vi "24_1.vi"() -> ()   [LabVIEW 2020]
panel:
  out "sum":i16=10
  in  "Switch":bool=TRUE
  in  "Input":string="nwneswnwnwsenwnwnwnwnwnwnwnwnwnenwnwnwnw\nseseswswseseswsesenwnwseseswsese\nswneeweneeneneeneeeeeneeeene\neswswnwswswwnwswswswswewswswswswswsw\nwwseneseeneseswwwseneseseneswseswese\nseseseswseseseseswnwswswneseseswsesesese\nnwnewwwwwswnwnwww\nneesenwwswseswswswnwsenwsesewseeeswse\nsweeneesweeswnweewseeneeneneswnw\nswseswseswswseseswseneswseswswsesesesese\nswneneneenenenenenenenenenenenwne\nswswswswswswswswswswswesenwseswswswse\nneeeenweneeneswene\nswwnenwsewwwswswwswwswweewwswwnw\nenewwnenwnenenenwnewnenenwnenenenwee\nnwwnwnwnwnwnwnwenewnwsenwwwwwnwswnw\neeenweeeesweeeneeseeeeswee\nwswwswseswwswswwwnww\nswenwwn..."
  in  "Input Test":string="sesenwnenenewseeswwswswwnenewsewsw\nneeenesenwnwwswnenewnwwsewnenwseswesw\nseswneswswsenwwnwse\nnwnwneseeswswnenewneswwnewseswneseene\nswweswneswnenwsewnwneneseenw\neesenwseswswnenwswnwnwsewwnwsene\nsewnenenenesenwsewnenwwwse\nwenwwweseeeweswwwnwwe\nwsweesenenewnwwnwsenewsenwwsesesenwne\nneeswseenwwswnwswswnw\nnenwswwsewswnenenewsenwsenwnesesenew\nenewnwewneswsewnwswenweswnenwsenwsw\nsweneswneswneneenwnewenewwneswswnese\nswwesenesewenwneswnwwneseswwne\nenesenwswwswneneswsenwnewswseenwsese\nwnwnesenesenenwwnenwsewesewsesesew\nnenewswnwewswnenesenwnesewesw\neneswnwswnwsenenwnwnwwseeswneewsenese\nneswnwewnwnwseenwseesewsenwsweewe\nwseweeenwnesenwwwswnew"
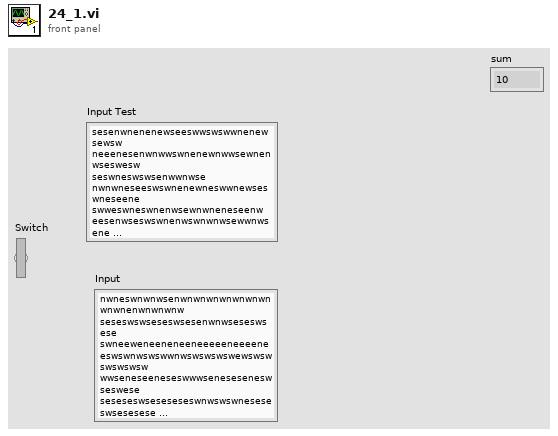
[diagram p1: front panel]
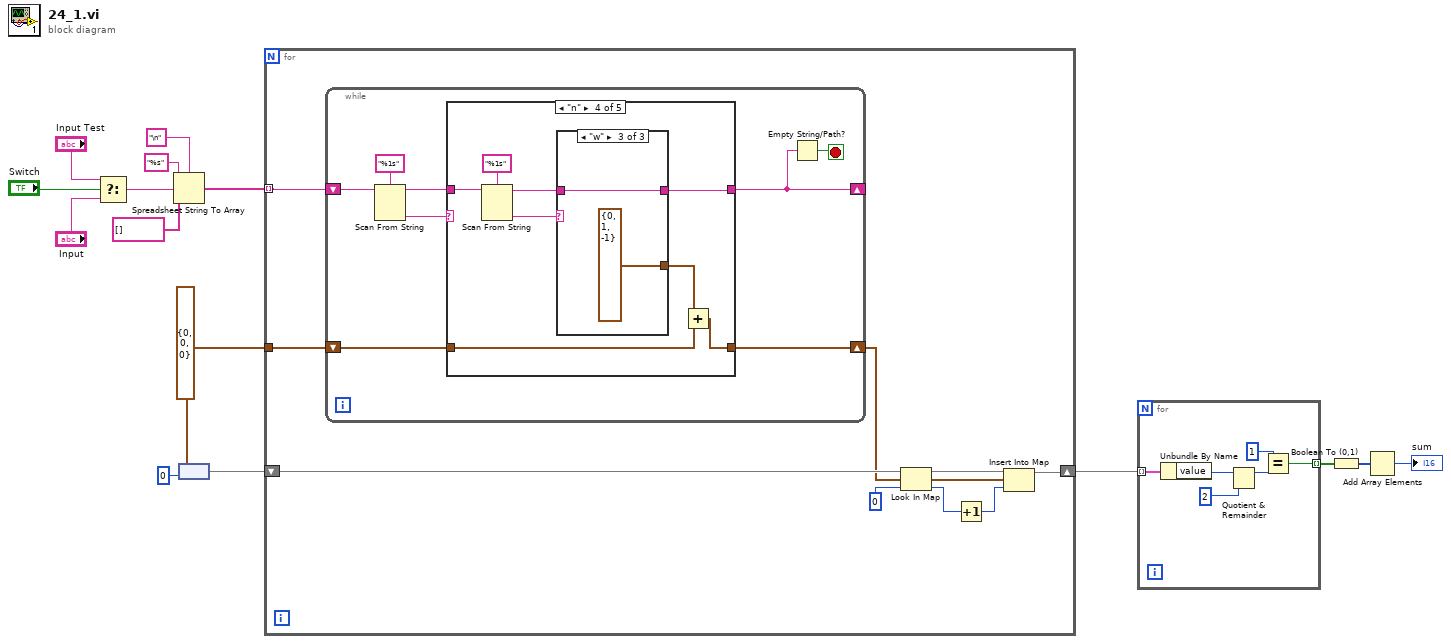
[diagram p0: block diagram]
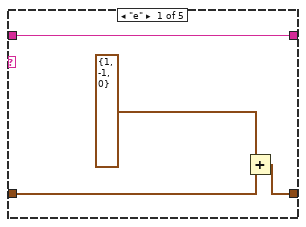
[diagram p2: hidden frame]
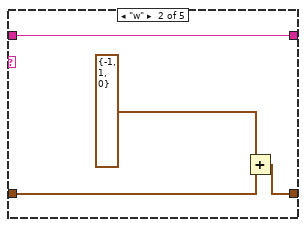
[diagram p3: hidden frame]
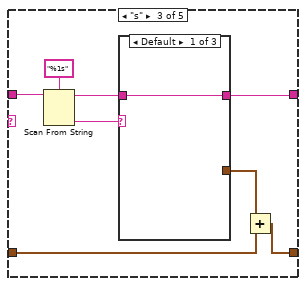
[diagram p4: hidden frame]
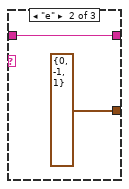
[diagram p5: hidden frame]
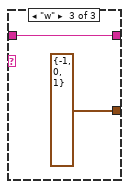
[diagram p6: hidden frame]
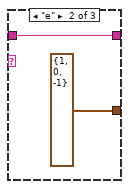
[diagram p8: hidden frame]
diagram:
  w7 = cluster{"x":i32, "y":i32, "z":i32} {"x"=0, "y"=0, "z"=0}
  n1 = Select(t="Input Test", s="Switch", f="Input") -> (s? t:f=w12:string)
  n2 = Spreadsheet String To Array(delimiter (Tab)="\n", format string="%s", spreadsheet string=w12, array type (2D Dbl)=string[] []) -> (array=w8:string[])
  n3 = node(w7, 0 ("value")) -> (w5:map{cluster{"x":i32, "y":i32, "z":i32}, i32})
  n4 = for {
    tunnel: w8 -> [w23] mode=indexing
    tunnel: w7 -> [w22]
    shift-right: [w16] -> w4
    shift-left: w5 -> [w20]
    n5 = while {
      shift-right: [w26] -> _
      shift-left: w23 -> [w31]
      shift-right: [w24] -> w19
      shift-left: w22 -> [w25]
      stop <- w29 stop-if-true
      n6 = Scan From String(format string="%1s", input string=w31) -> (remaining string=w27:string, output 1=w28:string)  [unwired: 3 in, 2 out]
      n7 = case shown="\"n\"" w28 {
        tunnel: w27 -> [w35 w39 w43 w56 w67]
        tunnel: [w35 w39 w41 w54 w67] -> w26
        tunnel: w25 -> [w32 w36 w45 w58 w66]
        tunnel: [w33 w37 w46 w59 w66] -> w24
        frame "e" {
          n8 = Add(x=cluster{"x":i32, "y":i32, "z":i32} {"x"=1, "y"=-1, "z"=0}, y=w32) -> (x+y=w33:cluster{"x":i32, "y":i32, "z":i32})
        }
        frame "w" {
          n9 = Add(x=cluster{"x":i32, "y":i32, "z":i32} {"x"=-1, "y"=1, "z"=0}, y=w36) -> (x+y=w37:cluster{"x":i32, "y":i32, "z":i32})
        }
        frame "s" {
          n10 = Scan From String(format string="%1s", input string=w43) -> (remaining string=w42:string, output 1=w40:string)  [unwired: 3 in, 2 out]
          n11 = case shown="Default" w40 {
            tunnel: [_ cluster{"x":i32, "y":i32, "z":i32} {"x"=0, "y"=-1, "z"=1} cluster{"x":i32, "y":i32, "z":i32} {"x"=-1, "y"=0, "z"=1}] -> w47
            tunnel: [w48 w49 w51] -> w41
            tunnel: w42 -> [w48 w49 w51]
            frame Default {
            }
            frame "e" {
            }
            frame "w" {
            }
          }
          n12 = Add(x=w47, y=w45) -> (x+y=w46:cluster{"x":i32, "y":i32, "z":i32})
        }
        frame "n" {
          n13 = Scan From String(format string="%1s", input string=w56) -> (remaining string=w55:string, output 1=w53:string)  [unwired: 3 in, 2 out]
          n14 = case shown="\"w\"" w53 {
            tunnel: [_ cluster{"x":i32, "y":i32, "z":i32} {"x"=1, "y"=0, "z"=-1} cluster{"x":i32, "y":i32, "z":i32} {"x"=0, "y"=1, "z"=-1}] -> w60
            tunnel: [w61 w62 w64] -> w54
            tunnel: w55 -> [w61 w62 w64]
            frame Default {
            }
            frame "e" {
            }
            frame "w" {
            }
          }
          n15 = Add(x=w60, y=w58) -> (x+y=w59:cluster{"x":i32, "y":i32, "z":i32})
        }
        frame Default {
        }
      }
      n16 = Empty String/Path?(string/path=w26) -> (empty?=w29:bool)
    }
    n17 = Look In Map(map=w20, key=w19, default value=0 ("value")) -> (value=w18:i32)  [unwired: 1 out]
    n18 = Increment(x=w18) -> (x+1=w17:i32)
    n19 = Insert Into Map(map in=w20, key=w19, value=w17) -> (map out=w16:map{cluster{"x":i32, "y":i32, "z":i32}, i32})  [unwired: 2 out]
  }
  n20 = for {
    tunnel: w4 -> [w73] mode=indexing
    tunnel: [w68] -> w3 mode=indexing
    n21 = Unbundle By Name(w73) -> ("value"=w72:i32)
    n22 = Quotient & Remainder(x=w72, y=2) -> (x-y*floor(x/y)=w70:i32)  [unwired: 1 out]
    n23 = Equal?(x=1, y=w70) -> (x = y?=w68:bool)
  }
  n24 = Boolean To (0,1)(Boolean=w3) -> (0, 1=w2:i16[])
  n25 = Add Array Elements(numeric array=w2) -> (sum=→"sum":i16)
